vi "Read Result String.vi"(11 "Method Result In":refnum<class "Method Result.lvclass">) -> (2 "Result String":string, 3 "Method Result Out":refnum<class "Method Result.lvclass">)   [LabVIEW 2020, in "Method Result.lvclass"]
uses:
  Method Result.lvclass
  Method Result.lvclass/Method Result.ctl
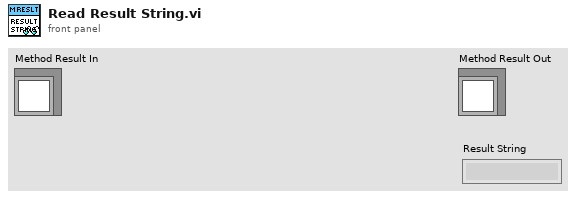
[diagram p1: front panel]
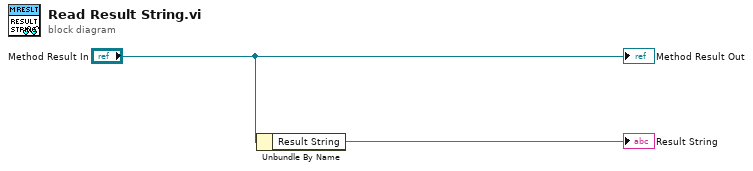
[diagram p0: block diagram]
diagram:
  n1 = Unbundle By Name("Method Result In") -> ("Result String"=→"Result String":string)
  "Method Result Out" <- "Method Result In"
